vi "InitConnection.vi"(8 "error in (no error)":errorcluster, 11 "Instrument in":refnum<class "Instrument.lvclass">) -> (0 "error out":errorcluster, 3 "Instrument out":refnum<class "Instrument.lvclass">)   [LabVIEW 2018, in "Instrument.lvclass"]
uses:
  Instrument.lvclass
  Server/Server.lvclass
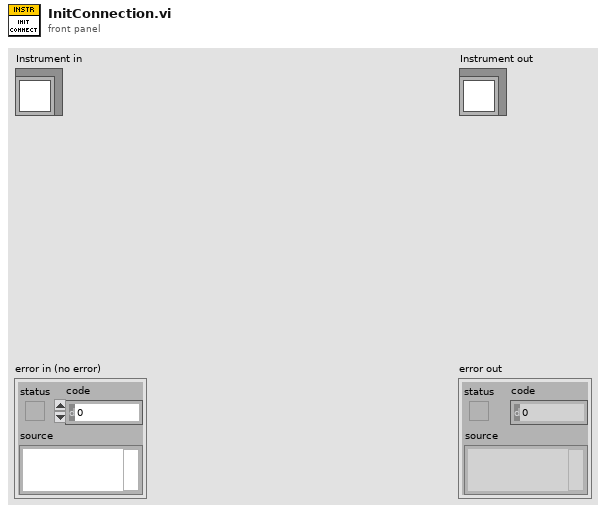
[diagram p1: front panel]
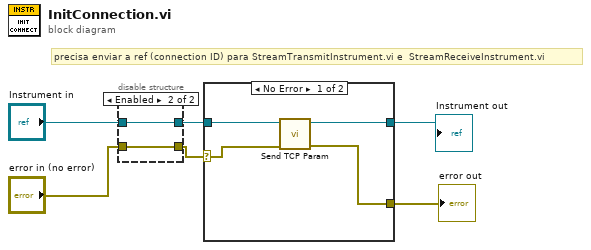
[diagram p0: block diagram]
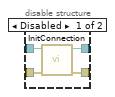
[diagram p2: hidden frame]
diagram:
  # "precisa enviar a ref (connection ID) para StreamTransmitInstrument.vi e  StreamReceiveInstrument.vi"
  n1 = disable-structure shown="Enabled" {
    disable-tunnel: "error in (no error)" -> [w10 w11]
    disable-tunnel: "Instrument in" -> [w9 w12]
    disable-tunnel: [w8 w12] -> w4
    disable-tunnel: [w7 w11] -> w3
    frame Disabled {
      n2 = call-parent "InitConnection.vi"("error in (no error)"=w10, "Server in"=w9) -> ("error out"=w7:errorcluster, "Server out"=w8:refnum<class "Instrument.lvclass">)  [unwired: 8 in]
    }
    frame Enabled {
    }
  }
  n3 = case shown="No Error" w3 {
    selector: w3 -> [w15 w17]
    tunnel: w4 -> [w16 w18]
    tunnel: [w14 w17] -> w2
    tunnel: [w13 w18] -> w1
    frame No Error {
      n4 = call-dynamic "Send TCP Param.vi"("error in (no error)"=w15, "Server in"=w16) -> ("error out"=w14:errorcluster, "Server out"=w13:refnum<class "Instrument.lvclass">)  [unwired: 8 in]
    }
    frame Error {
    }
  }
  "error out" <- w2
  "Instrument out" <- w1
